vi "point-by-point speed and angle with torque filter.vi"(6 "encoders offset":u32 caption="encoder offset @ 1Hz (ticks)", 8 "speed history in":u32[](array[numeric])=[0, 0, 0, 0, 0, 0, 0, 0, 0, 0, 0, 0, 0, 0, 0, 0, 0, 0, 0, 0, 0, 0, 0, 0, 0, 0, 0, 0, 0, 0, 0, 0, 0, 0, 0, 0, 0, 0, 0, 0], 9 "torque history":i32[](array[numeric])=[0, 0, 0, 0, 0, 0, 0, 0, 0, 0, 0, 0, 0, 0, 0, 0, 0, 0, 0, 0, 0, 0, 0, 0, 0, 0, 0, 0, 0, 0, 0, 0, 0, 0, 0, 0, 0, 0, 0, 0], 10 "angle pulse":u32, 11 "speed pulse":u32) -> (0 "speed history out":u32[](array[numeric]), 1 "torque history out":i32[](array[numeric]), 2 "calculated angle (degrees)":sgl, 3 "calculated speed (Hz)":sgl, 4 "measured encoder delta":sgl)   [LabVIEW 2018]
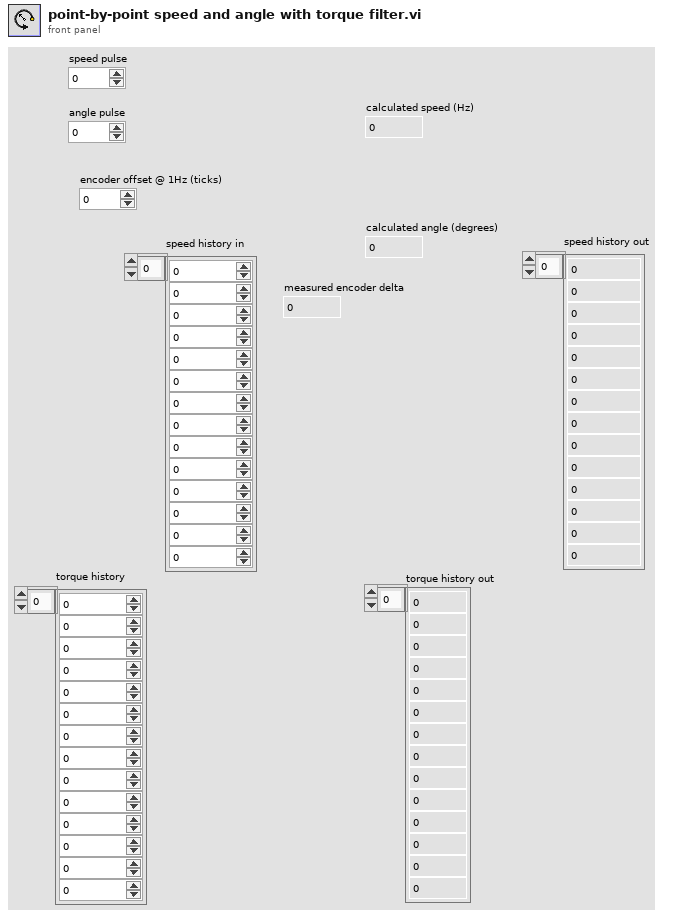
[diagram p1: front panel]
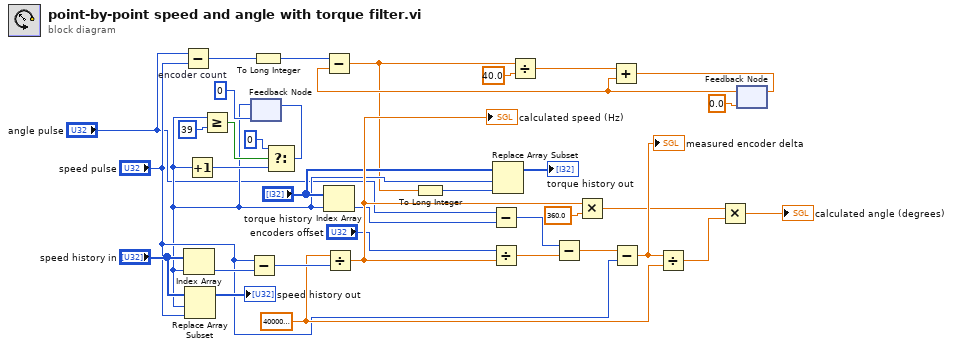
[diagram p0: block diagram]
diagram:
  w20 = 0  # encoder count
  w31 = sgl 40000000.0 ("64bit integer")
  n1 = Subtract(x="angle pulse", y="speed pulse") -> (x-y=w7:u32)
  n2 = feedback #1(w20) -> (w8:i32)
  n3 = Index Array(array="speed history in", index=w8) -> (element=w36:u32)
  n4 = Replace Array Subset(array="speed history in", new element="speed pulse", index=w8) -> (→"speed history out":u32[])
  n5 = Increment(x=w8) -> (x+1=w22:i32)
  n6 = Greater Or Equal?(x=w8, y=39) -> (x >= y?=w23:bool)
  n7 = Subtract(x="speed pulse", y=w36) -> (x-y=w35:u32)
  n8 = To Long Integer(number=w7) -> (32bit integer=w14:i32)
  n9 = Select(t=0, s=w23, f=w22) -> (s? t:f=w19:i32)
  n10 = feedback-in #1(w19) -> ()
  n11 = Index Array(array="torque history", index=w8) -> (element=w4:i32)
  n12 = Divide(x=w31, y=w35) -> (x/y=w26:sgl)
  "calculated speed (Hz)" <- w26
  n13 = Subtract(x="angle pulse", y=w4) -> (x-y=w3:u32)
  n14 = Divide(x="encoders offset", y=w26) -> (x/y=w27:sgl)
  n15 = Subtract(x=w3, y=w27) -> (x-y=w34:sgl)
  n16 = Multiply(x=w26, y=sgl 360.0) -> (x*y=w29:sgl)
  n17 = Subtract(x=w34, y="speed pulse") -> (x-y=w32:sgl)
  "measured encoder delta" <- w32
  n18 = Divide(x=w32, y=w31) -> (x/y=w30:sgl)
  n19 = Multiply(x=w29, y=w30) -> (x*y=→"calculated angle (degrees)":sgl)
  n20 = feedback #2(sgl 0.0) -> (w11:sgl)
  n21 = Subtract(x=w14, y=w11) -> (x-y=w6:sgl)
  n22 = To Long Integer(number=w6) -> (32bit integer=w1:i32)
  n23 = Replace Array Subset(array="torque history", new element=w1, index=w8) -> (→"torque history out":i32[])
  n24 = Divide(x=w6, y=sgl 40.0) -> (x/y=w13:sgl)
  n25 = Add(x=w13, y=w11) -> (x+y=w12:sgl)
  n26 = feedback-in #2(w12) -> ()
